vi "Get Screen Header Data.vi"(8 "error in":errorcluster, 11 "VISA session":refnum<visa-resource-name>) -> (0 "error out":errorcluster, 2 "Head JSON":string, 3 "VISA session out":refnum<visa-resource-name>)   [LabVIEW 2023, in "OWON SDS1022.lvlib"]
uses:
  OWON SDS1022.lvlib
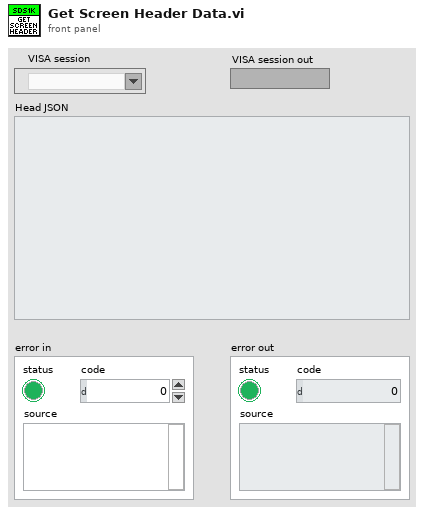
[diagram p1: front panel]
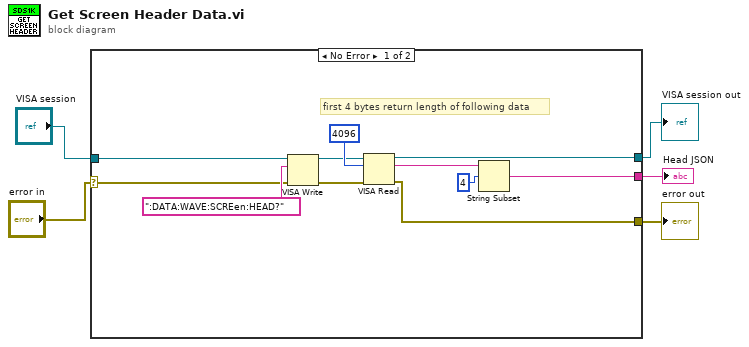
[diagram p0: block diagram]
diagram:
  n1 = case shown="No Error" "error in" {
    selector: "error in" -> [w12 w17]
    tunnel: [w6 _] -> w1
    tunnel: "VISA session" -> [w11 w18]
    tunnel: [w8 w18] -> w3
    tunnel: [w7 w17] -> w2
    frame No Error {
      # "first 4 bytes return length of following data"
      n2 = VISA Write(VISA resource name=w11, write buffer=":DATA:WAVE:SCREen:HEAD?", error in (no error)=w12) -> (VISA resource name out=w13:refnum<visa-resource-name>, error out=w14:errorcluster)  [unwired: 1 out]
      n3 = VISA Read(VISA resource name=w13, byte count=u32 4096, error in (no error)=w14) -> (VISA resource name out=w8:refnum<visa-resource-name>, read buffer=w10:string, error out=w7:errorcluster)  [unwired: 1 out]
      n4 = String Subset(string=w10, offset (0)=4) -> (substring=w6:string)  [unwired: 1 in]
    }
    frame Error {
    }
  }
  "VISA session out" <- w3
  "error out" <- w2
  "Head JSON" <- w1
